vi "Timing Sequence to Fiber Triggers Cluster (conflict at 2013-06-19_20-52-24).vi"(8 "Timing Sequence 2":T2(array[cluster]), 11 "Timing Sequence":T2(array[cluster])) -> (0 "Fiber Triggers 2":T1(array[cluster])=[{"[actual delay (s)]"=0.003, "[actual width (s)]"=0.005, "Active"=TRUE, "Channel Name"="Puff 1", "counter"="PXI1Slot9/ctr0"}, {"[actual delay (s)]"=0.001, "[actual width (s)]"=0.5, "Active"=TRUE, "Channel Name"="Puff 2", "counter"="PXI1Slot9/ctr1"}, {"[actual delay (s)]"=0.0003, "[actual width (s)]"=0.0004, "Active"=FALSE, "Channel Name"="Puff 3", "counter"="PXI1Slot9/ctr2"}, {"[actual delay (s)]"=0.0005, "[actual width (s)]"=0.0004, "Active"=FALSE, "Channel Name"="Puff 4", "counter"="PXI1Slot9/ctr3"}, {"[actual delay (s)]"=0.001, "[actual width (s)]"=0.5, "Active"=FALSE, "Channel Name"="Open", "counter"="PXI1Slot9/ctr4"}, {"[actual delay (s)]"=0.001, "[actual width (s)]"=0.5, "Active"=FALSE, "Channel Name"="Open", "counter"="PXI1Slot9/ctr5"}, {"[actual delay (s)]"=0.001, "[actual width (s)]"=0.5, "Active"=FALSE, "Channel Name"="Open", "counter"="PXI1Slot9/ctr6"}, {"[actual delay (s)]"=0.001, "[actual width (s)]"=0.5, "Active"=FALSE, "Channel Name"="Open", "counter"="PXI1Slot9/ctr7"}] {"[actual width (s)]" format="%.3p"; "[actual delay (s)]" format="%.3p"}, 3 "Fiber Triggers":T1(array[cluster])=[{"[actual delay (s)]"=0.001, "[actual width (s)]"=0.5, "Active"=TRUE, "Channel Name"="Gun B1", "counter"="PXI1Slot8/ctr0"}, {"[actual delay (s)]"=0.001, "[actual width (s)]"=0.5, "Active"=TRUE, "Channel Name"="Gun B2", "counter"="PXI1Slot8/ctr1"}, {"[actual delay (s)]"=0.001, "[actual width (s)]"=0.5, "Active"=TRUE, "Channel Name"="Gun B3", "counter"="PXI1Slot8/ctr2"}, {"[actual delay (s)]"=0.001, "[actual width (s)]"=0.5, "Active"=TRUE, "Channel Name"="Sol B1", "counter"="PXI1Slot8/ctr3"}, {"[actual delay (s)]"=0.001, "[actual width (s)]"=0.5, "Active"=TRUE, "Channel Name"="Sol B2", "counter"="PXI1Slot8/ctr4"}, {"[actual delay (s)]"=0.001, "[actual width (s)]"=0.5, "Active"=TRUE, "Channel Name"="Sol B3", "counter"="PXI1Slot8/ctr5"}, {"[actual delay (s)]"=0.001, "[actual width (s)]"=0.5, "Active"=FALSE, "Channel Name"="Open", "counter"="PXI1Slot8/ctr6"}, {"[actual delay (s)]"=0.003, "[actual width (s)]"=0.0002, "Active"=FALSE, "Channel Name"="Open", "counter"="PXI1Slot8/ctr7"}] {"[actual width (s)]" format="%1.3p"; "[actual delay (s)]" format="%.3p"})   [LabVIEW 2012]
doc: "Converts timing sequence cluster into Preexisting Fiber Trigger cluster\nTimes are converted to seconds. Delay Times are changed from relative reference to absolute reference.\n\nExample:\ntime: -10 --> 0\ntime: -5 --> 5\ntime: 0 --> 10\ntime: 3 --> 13"
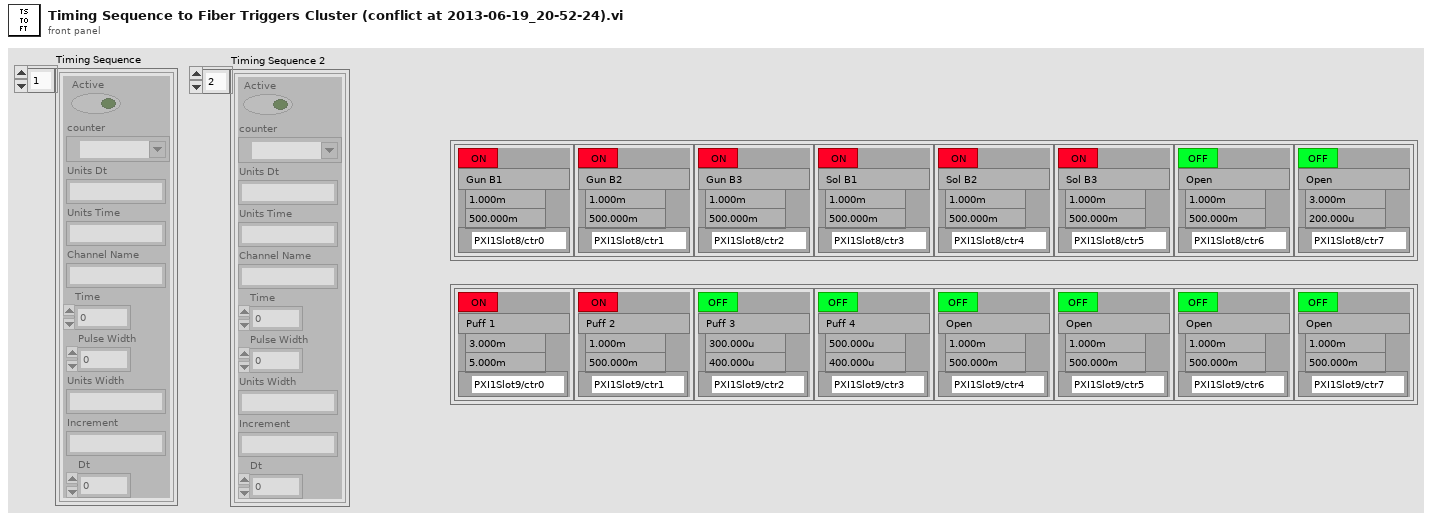
[diagram p1: front panel]
types:
  T1 = cluster{"[actual delay (s)]":dbl, "[actual width (s)]":dbl, "Active":bool, "Channel Name":string, "counter":tag}[]
  T2 = cluster{"Active":bool, "counter":tag, "Units Dt":string, "Units Time":string, "Channel Name":string, "Time":dbl, "Pulse Width":dbl, "Units Width":string, "Increment":string, "Dt":dbl}[]
  T3 = cluster{"[actual delay (s)]":dbl, "[actual width (s)]":dbl, "Active":bool, "Channel Name":string, "counter":tag}
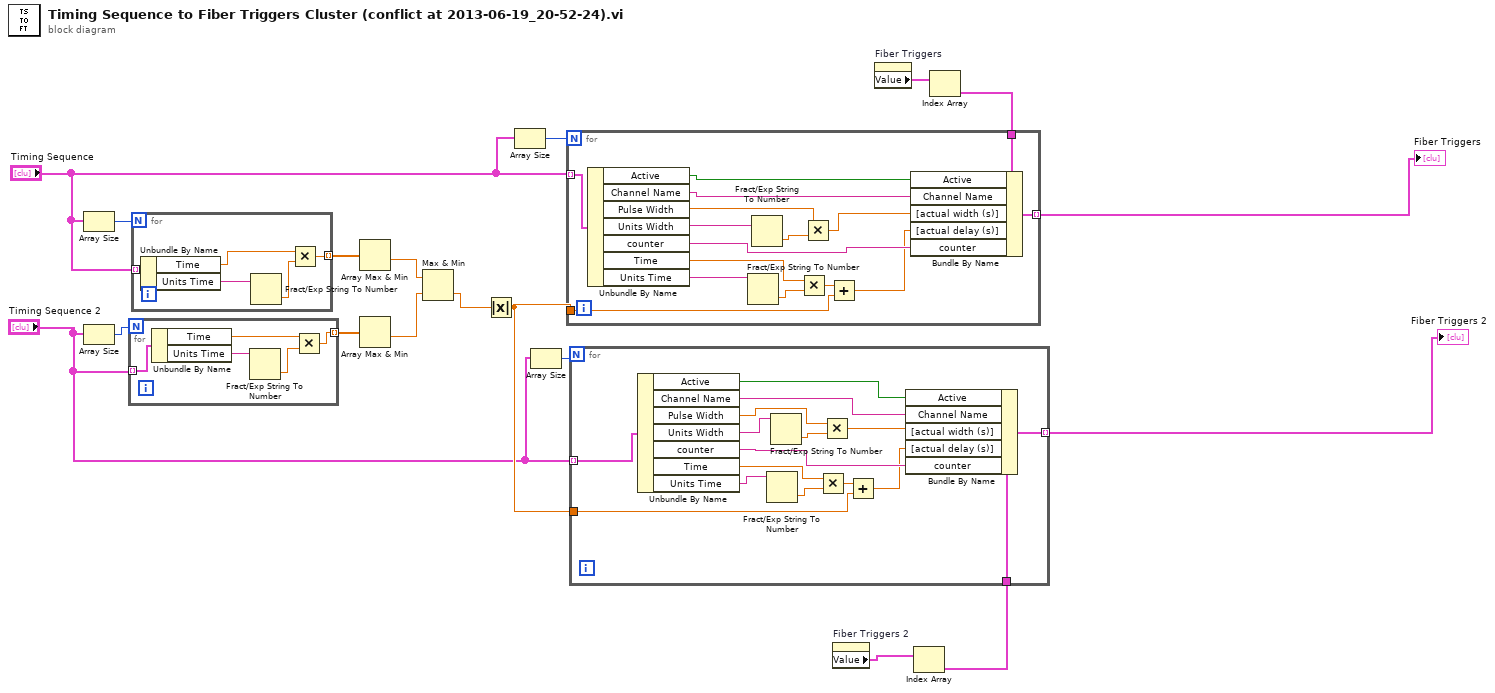
[diagram p0: block diagram]
diagram:
  n1 = Array Size(array="Timing Sequence") -> (size(s)=w13:i32)
  n2 = Array Size(array="Timing Sequence 2") -> (size(s)=w9:i32)
  n3 = for {
    N: w9 -> [_]
    tunnel: [w20] -> w10 mode=indexing
    tunnel: "Timing Sequence 2" -> [w19] mode=indexing
    n4 = Unbundle By Name(w19) -> ("Time"=w22:dbl, "Units Time"=w23:string)
    n5 = Fract/Exp String To Number(string=w23) -> (number=w21:dbl)  [unwired: 3 in, 1 out]
    n6 = Multiply(x=w22, y=w21) -> (x*y=w20:dbl)
  }
  n7 = for {
    N: w13 -> [_]
    tunnel: "Timing Sequence" -> [w28] mode=indexing
    tunnel: [w24] -> w18 mode=indexing
    n8 = Unbundle By Name(w28) -> ("Time"=w25:dbl, "Units Time"=w27:string)
    n9 = Fract/Exp String To Number(string=w27) -> (number=w26:dbl)  [unwired: 3 in, 1 out]
    n10 = Multiply(x=w25, y=w26) -> (x*y=w24:dbl)
  }
  n11 = Array Max & Min(array=w18) -> (min value=w15:dbl)  [unwired: 3 out]
  n12 = Array Max & Min(array=w10) -> (min value=w16:dbl)  [unwired: 3 out]
  n13 = Max & Min(x=w15, y=w16) -> (min(x,y)=w14:dbl)  [unwired: 1 out]
  n14 = Absolute Value(x=w14) -> (abs(x)=w8:dbl)
  n15 = Array Size(array="Timing Sequence") -> (size(s)=w12:i32)
  n16 = Array Size(array="Timing Sequence 2") -> (size(s)=w6:i32)
  n17 = property on="Fiber Triggers 2" class="Arr (strict)"() -> ("Value"=w2:T1)  [unwired: 2 in, 2 out]
  n18 = property on="Fiber Triggers" class="Arr (strict)"() -> ("Value"=w4:T1)  [unwired: 2 in, 2 out]
  n19 = Index Array(array=w2) -> (element=w1:T3)  [unwired: 1 in]
  n20 = for {
    N: w6 -> [_]
    tunnel: w8 -> [w32]
    tunnel: w1 -> [w31]
    tunnel: [w30] -> w7 mode=indexing
    tunnel: "Timing Sequence 2" -> [w29] mode=indexing
    n21 = Unbundle By Name(w29) -> ("Active"=w33:bool, "Channel Name"=w34:string, "Pulse Width"=w41:dbl, "Units Width"=w40:string, "counter"=w37:tag, "Time"=w39:dbl, "Units Time"=w38:string)
    n22 = Fract/Exp String To Number(string=w38) -> (number=w43:dbl)  [unwired: 3 in, 1 out]
    n23 = Fract/Exp String To Number(string=w40) -> (number=w44:dbl)  [unwired: 3 in, 1 out]
    n24 = Multiply(x=w39, y=w43) -> (x*y=w42:dbl)
    n25 = Multiply(x=w41, y=w44) -> (x*y=w35:dbl)
    n26 = Add(x=w42, y=w32) -> (x+y=w36:dbl)
    n27 = Bundle By Name(cluster=w31, "Active"=w33, "Channel Name"=w34, "[actual width (s)]"=w35, "[actual delay (s)]"=w36, "counter"=w37) -> (w30:T3)
  }
  "Fiber Triggers 2" <- w7
  n28 = Index Array(array=w4) -> (element=w3:T3)  [unwired: 1 in]
  n29 = for {
    N: w12 -> [_]
    tunnel: "Timing Sequence" -> [w60] mode=indexing
    tunnel: w8 -> [w46]
    tunnel: [w47] -> w17 mode=indexing
    tunnel: w3 -> [w45]
    n30 = Unbundle By Name(w60) -> ("Active"=w59:bool, "Channel Name"=w58:string, "Pulse Width"=w56:dbl, "Units Width"=w57:string, "counter"=w53:tag, "Time"=w51:dbl, "Units Time"=w52:string)
    n31 = Fract/Exp String To Number(string=w52) -> (number=w50:dbl)  [unwired: 3 in, 1 out]
    n32 = Fract/Exp String To Number(string=w57) -> (number=w55:dbl)  [unwired: 3 in, 1 out]
    n33 = Multiply(x=w51, y=w50) -> (x*y=w49:dbl)
    n34 = Multiply(x=w56, y=w55) -> (x*y=w54:dbl)
    n35 = Add(x=w49, y=w46) -> (x+y=w48:dbl)
    n36 = Bundle By Name(cluster=w45, "Active"=w59, "Channel Name"=w58, "[actual width (s)]"=w54, "[actual delay (s)]"=w48, "counter"=w53) -> (w47:T3)
  }
  "Fiber Triggers" <- w17
